vi "StRtMotionto0-Home.vi"(8 "error in (no error)":errorcluster, 9 "Axis (1..4)":T1=1 items=["X"=1, "Y"=2, "Z"=3, "T"=4], 11 "VXMx2 in":refnum<class "VXMx2.lvclass">) -> (0 "error out":errorcluster, 3 "VXMx2 out":refnum<class "VXMx2.lvclass">)   [LabVIEW 2019, in "VXMx2.lvclass"]
doc: "for a give subset object, start one axis moving to home, absolute 0 motor position.\n this command implemented:\nIAmM0 Index motor to Absolute zero position, m=motor# (1,2,3,4)"
uses:
  VXMx2.lvclass
  <instrlib>/Velmex VXM/Public/VXM Axis.ctl
  VXMx2.lvclass/VXMx2.ctl
  <instrlib>/Velmex VXM/Velmex VXM.lvlib
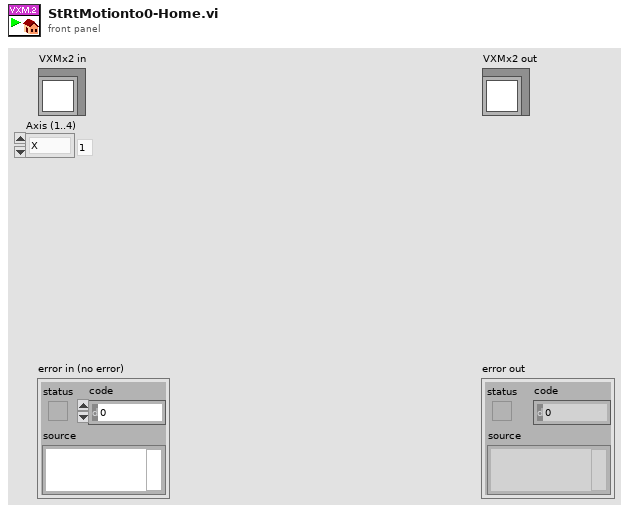
[diagram p1: front panel]
types:
  T1 = typedef "Velmex VXM.lvlib/VXM Axis.ctl" = u16
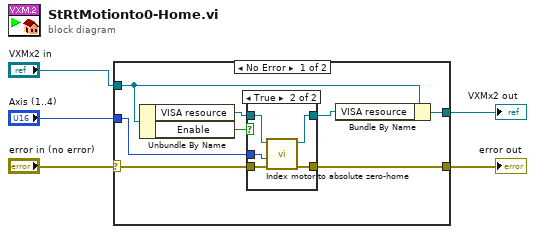
[diagram p0: block diagram]
diagram:
  n1 = case shown="No Error" "error in (no error)" {
    selector: "error in (no error)" -> [w10 w22]
    tunnel: [w9 w22] -> w2
    tunnel: [w13 w21] -> w1
    tunnel: "VXMx2 in" -> [w7 w21]
    tunnel: "Axis (1..4)" -> [w6 _]
    frame No Error {
      n2 = Unbundle By Name(w7) -> ("VISA resource"=w12:refnum<visa-resource-name>, "Enable"=w8:bool)
      n3 = case shown="True" w8 {
        tunnel: w12 -> [w15 w20]
        tunnel: [w15 w19] -> w11
        tunnel: w10 -> [w14 w18]
        tunnel: [w14 w17] -> w9
        tunnel: w6 -> [_ w16]
        frame False {
        }
        frame True {
          n4 = call <instrlib>:"Index motor to absolute zero-home.vi"("error in (no error)"=w18, "Axis (1..4)"=w16, "VISA resource name"=w20) -> ("error out"=w17:errorcluster, "VISA resource out"=w19:refnum<visa-resource-name>)  [unwired: 7 in]
        }
      }
      n5 = Bundle By Name(cluster=w7, "VISA resource"=w11) -> (w13:refnum<class "VXMx2.lvclass">)
    }
    frame Error {
    }
  }
  "error out" <- w2
  "VXMx2 out" <- w1
